vi "Find Named Range.vi"(8 "error in":errorcluster, 10 "Range Identifier":string, 11 "OpenXml in":refnum<class "OpenXml.lvclass">) -> (0 "error out":errorcluster, 1 "End Cell":cluster{"Col":string, "Row":i32}, 2 "Start Cell":cluster{"Col":string, "Row":i32}, 3 "OpenXml out":refnum<class "OpenXml.lvclass">)   [LabVIEW 2024, in "OpenXml.lvclass"]
uses:
  OpenXml.lvclass
  OpenXml.lvclass/OpenXml.ctl
  C:/Users/tupp_js/.nuget/packages/documentformat.openxml/3.3.0/lib/net46/DocumentFormat.OpenXml.dll
  .nuget/packages/documentformat.openxml/3.3.0/lib/net46/DocumentFormat.OpenXml.dll
  C:/Users/tupp_js/Documents/LabVIEW Data/OpenXml LabVIEW/DocumentFormat.OpenXml.Framework.dll
  DocumentFormat.OpenXml.Framework.dll
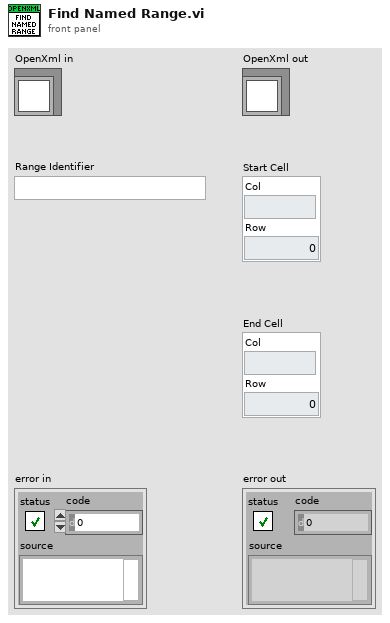
[diagram p1: front panel]
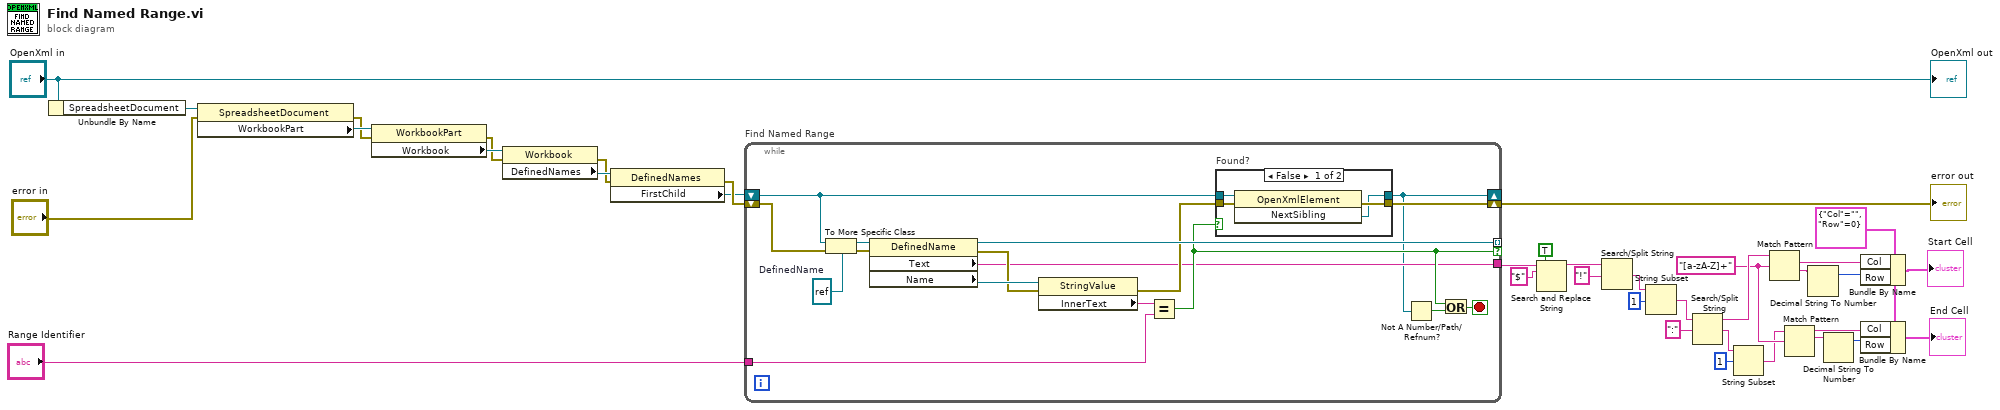
[diagram p0: block diagram]
diagram:
  w6 = cluster{"Col":string, "Row":i32} {"Col"="", "Row"=0} ("input cluster")
  w8 = "[a-zA-Z]+" ("regular expression")
  n1 = Unbundle By Name("OpenXml in") -> ("SpreadsheetDocument"=w35:refnum<k24>)
  n2 = property class="SpreadsheetDocument"(reference=w35, error in="error in") -> (error out=w28:errorcluster, "WorkbookPart"=w33:refnum<k24>)  [unwired: 1 out]
  n3 = property class="WorkbookPart"(reference=w33, error in=w28) -> (error out=w27:errorcluster, "Workbook"=w34:refnum<k24>)  [unwired: 1 out]
  n4 = property class="Workbook"(reference=w34, error in=w27) -> (error out=w26:errorcluster, "DefinedNames"=w32:refnum<k24>)  [unwired: 1 out]
  n5 = property class="DefinedNames"(reference=w32, error in=w26) -> (error out=w31:errorcluster, "FirstChild"=w24:refnum<k24>)  [unwired: 1 out]
  n6 = while "Find Named Range" {
    shift-right: [w47] -> w25
    shift-left: w31 -> [w53]
    tunnel: [w49] -> _ mode=indexing if=w42
    tunnel: "Range Identifier" -> [w44]
    tunnel: [w39] -> w21
    shift-right: [w37] -> _
    shift-left: w24 -> [w38]
    stop <- w51 stop-if-true
    w41 = refnum<k24> refnum  # DefinedName
    n7 = To More Specific Class(target class=w41, reference=w38, error in=w53) -> (specific class reference=w50:refnum<k24>, error out=w48:errorcluster)
    n8 = property class="DefinedName"(reference=w50, error in=w48) -> (reference out=w49:refnum<k24>, error out=w45:errorcluster, "Text"=w39:string, "Name"=w46:refnum<k24>)
    n9 = property class="StringValue"(reference=w46, error in=w45) -> (error out=w43:errorcluster, "InnerText"=w40:string)  [unwired: 1 out]
    n10 = Equal?(x=w40, y=w44) -> (x = y?=w42:bool)
    n11 = case "Found?" shown="False" w42 {
      tunnel: [w57 w59] -> w47
      tunnel: w38 -> [w56 w58]
      tunnel: w43 -> [w55 w59]
      tunnel: [w54 w58] -> w37
      frame False {
        n12 = invoke class="OpenXmlElement" method="NextSibling"(reference=w56, error in=w55) -> (error out=w57:errorcluster, "NextSibling"=w54:refnum<k24>)  [unwired: 1 in, 1 out]
      }
      frame True {
      }
    }
    n13 = Not A Number/Path/Refnum?(number/path/refnum=w37) -> (NaN/Path/Refnum?=w52:bool)
    n14 = Or(x=w42, y=w52) -> (x .or. y?=w51:bool)
  }
  "error out" <- w25
  n15 = Search and Replace String(replace all?=TRUE ("replace all? (F)"), input string=w21, search string="$") -> (result string=w19:string)  [unwired: 5 in, 3 out]
  n16 = Search/Split String(string=w19, search string/char (-)="!") -> (match + rest of string=w17:string)  [unwired: 1 in, 2 out]
  n17 = String Subset(string=w17, offset (0)=1) -> (substring=w15:string)  [unwired: 1 in]
  n18 = Search/Split String(string=w15, search string/char (-)=":") -> (substring before match=w12:string, match + rest of string=w13:string)  [unwired: 1 in, 1 out]
  n19 = String Subset(string=w13, offset (0)=1) -> (substring=w7:string)  [unwired: 1 in]
  n20 = Match Pattern(string=w12, regular expression=w8) -> (match substring=w11:string, after substring=w10:string)  [unwired: 1 in, 2 out]
  n21 = Match Pattern(string=w7, regular expression=w8) -> (before substring=w3:string, match substring=w2:string)  [unwired: 1 in, 2 out]
  n22 = Decimal String To Number(string=w10) -> (offset past number=w9:i32)  [unwired: 2 in, 1 out]
  n23 = Decimal String To Number(string=w2) -> (offset past number=w1:i32)  [unwired: 2 in, 1 out]
  n24 = Bundle By Name(cluster=w6, "Col"=w11, "Row"=w9) -> (→"Start Cell":cluster{"Col":string, "Row":i32})
  n25 = Bundle By Name(cluster=w6, "Col"=w3, "Row"=w1) -> (→"End Cell":cluster{"Col":string, "Row":i32})
  "OpenXml out" <- "OpenXml in"
